vi "Disable All Loggers.vi"(8 "error in":errorcluster) -> (0 "error out":errorcluster)   [LabVIEW 2018, in "GLog.lvlib"]
uses:
  GLog.lvlib
  registry/Registry.lvlib
panel:
  # "Connector Pane"
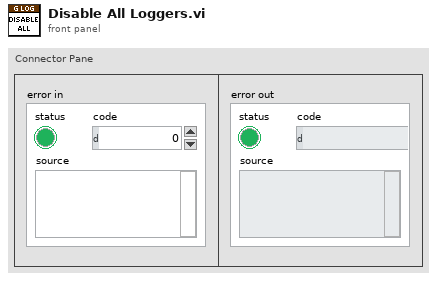
[diagram p1: front panel]
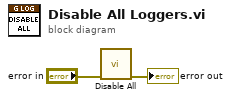
[diagram p0: block diagram]
diagram:
  n1 = call "Disable All.vi"("error in"="error in") -> ("error out"=→"error out":errorcluster)  [unwired: 10 in]
